vi "Helper SubVI - Signal Sweep (tfa).vi"(7 "reset":bool, 9 "length":i32=-1, 10 "shift (%)":dbl=25.0, 11 "Signal in":dbl[](array[numeric])) -> (3 "Signal out":dbl[](array[numeric]))   [LabVIEW 2023]
doc: "Rotates the signal or gets a subset from the input signal."
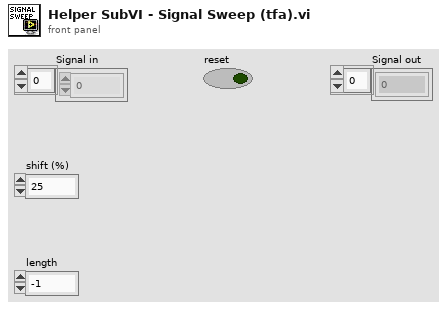
[diagram p1: front panel]
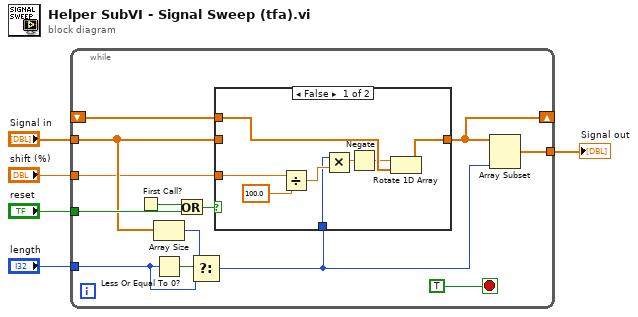
[diagram p0: block diagram]
diagram:
  n1 = while {
    shift-right: [w11] -> _
    shift-left: _ -> [w15]
    tunnel: "reset" -> [w10]
    tunnel: "Signal in" -> [w9]
    tunnel: "length" -> [w8]
    tunnel: "shift (%)" -> [w7]
    tunnel: [w6] -> w1
    stop <- TRUE stop-if-true
    n2 = First Call?() -> (First Call?: T/F=w18:bool)
    n3 = Array Size(array=w9) -> (size(s)=w13:i32)
    n4 = Less Or Equal To 0?(x=w8) -> (x <= 0?=w14:bool)
    n5 = Or(x=w18, y=w10) -> (x .or. y?=w17:bool)
    n6 = Select(t=w13, s=w14, f=w8) -> (s? t:f=w12:i32)
    n7 = case shown="False" w17 {
      tunnel: w9 -> [_ w27]
      tunnel: [w26 w27] -> w11
      tunnel: w15 -> [w23 _]
      tunnel: w12 -> [w20 _]
      tunnel: w7 -> [w19 _]
      frame False {
        n8 = Divide(x=w19, y=100.0) -> (x/y=w25:dbl)
        n9 = Multiply(x=w20, y=w25) -> (x*y=w22:dbl)
        n10 = Negate(x=w22) -> (-x=w21:dbl)
        n11 = Rotate 1D Array(1:w23, 2:w21) -> (0:w26:dbl[])
      }
      frame True {
      }
    }
    n12 = Array Subset(array=w11, length=w12) -> (w6:dbl[])  [unwired: 1 in]
  }
  "Signal out" <- w1
